vi "prechirper tester.vi"() -> ()   [LabVIEW 2017]
uses:
  Serial Comms/Visa resource.ctl
  Prechirper control/Prechirper commands.ctl
panel:
  out "number":dbl
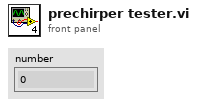
[diagram p1: front panel]
types:
  T1 = typedef "Prechirper commands.ctl" = enum16{"Prism 1 read", "Prism 1 set", "Prism 2 read", "Prism 2 set", "Wavelength read", "Wavelength Femto set", "Wavelength Femto and Laser set", "GVD curve number read", "GVD curve number set"}
  T2 = typedef "Visa resource.ctl" = cluster{"VISA resource name":refnum<visa-resource-name>, "baud rate":u32}
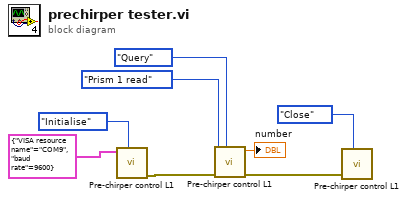
[diagram p0: block diagram]
diagram:
  n1 = call "Pre-chirper control L1.vi"("State"=enum16{"Initialise", "Query", "Close"}."Initialise", "Visa resource"=T2 {"VISA resource name"="COM9", "baud rate"=9600}) -> ("error out"=w6:errorcluster)  [unwired: 8 in, 1 out]
  n2 = call "Pre-chirper control L1.vi"("State"=enum16{"Initialise", "Query", "Close"}."Query", "error in (no error)"=w6, "Pre-chirper commands"=Prechirper_commands."Prism 1 read") -> ("error out"=w2:errorcluster, "number"=→"number":dbl)  [unwired: 7 in]
  n3 = call "Pre-chirper control L1.vi"("State"=enum16{"Initialise", "Query", "Close"}."Close", "error in (no error)"=w2) -> ()  [unwired: 8 in, 2 out]
